vi "MotorSimulation.vi"() -> ()   [LabVIEW 2022 SP3]
panel:
  out "Input and theta":cluster{"Signal Gen":dbl, "Thetadot Out":dbl}(graph)
  in  "System Parameters":cluster{"a1":dbl, "a0":dbl, "a2 ":dbl, "b":dbl}={"a1"=0.1894, "a0"=0.0, "a2 "=0.0052, "b"=0.3334}
  in  "Ring":u16(ring) items=["square", "triangle", "sinusoidal"]
  in  "stop":bool
  out "Input and thetadot":cluster{"Signal Gen":dbl, "Thetadot Out":dbl}(graph)
  in  "Amplitude":dbl
  in  "Signal Freq (Hz)":dbl
  in  "Sampling Time  (s)":dbl
  # "Lab 2"
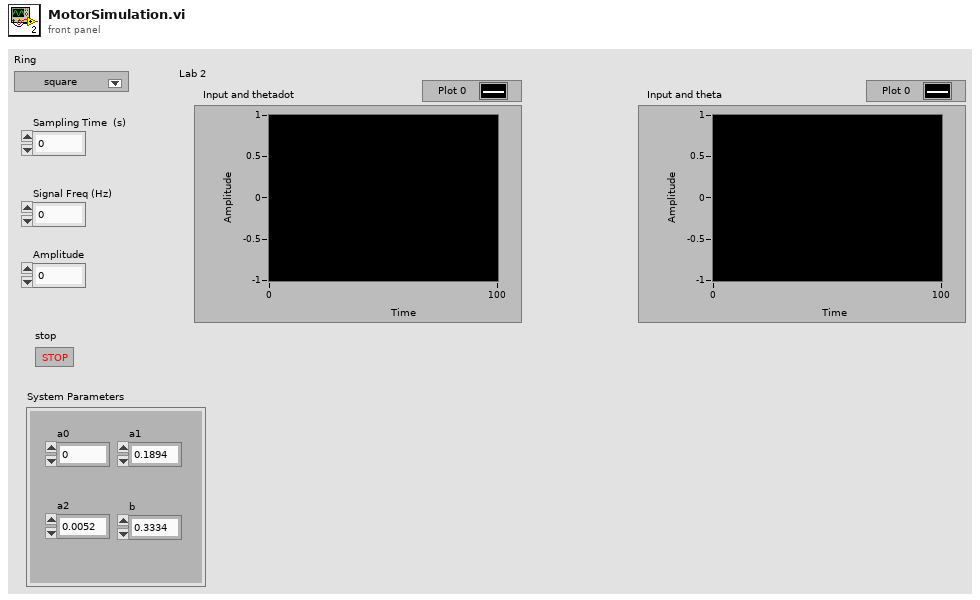
[diagram p1: front panel]
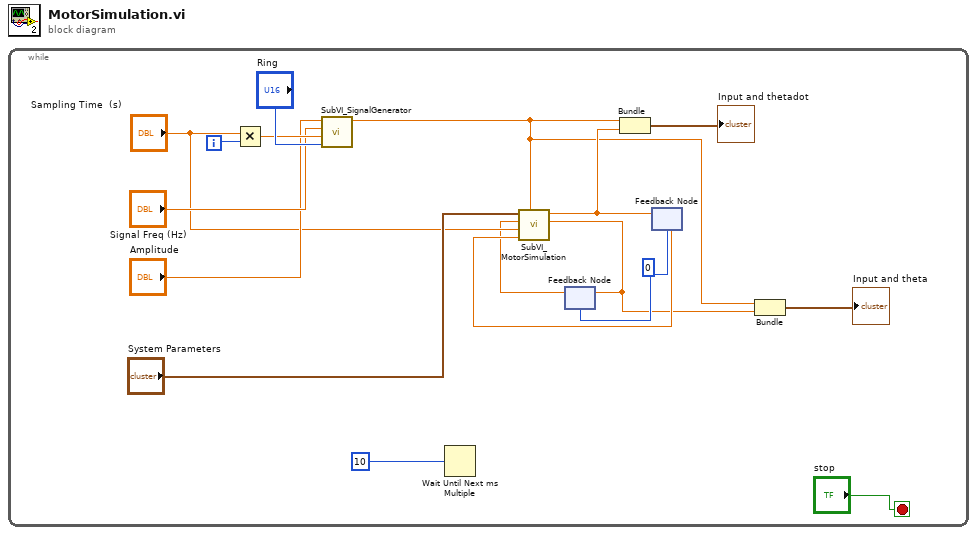
[diagram p0: block diagram]
diagram:
  n1 = while {
    i -> [w15]
    stop <- "stop" stop-if-true
    w7 = 0
    n2 = Multiply(x="Sampling Time  (s)", y=w15) -> (x*y=w14:dbl)
    n3 = call "SubVI_SignalGenerator.vi"("Signal Type"="Ring", "Time"=w14, "Freq"="Signal Freq (Hz)", "Amplitude"="Amplitude") -> ("Signal Gen"=w4:dbl)  [unwired: 7 in]
    n4 = Wait Until Next ms Multiple(millisecond multiple=10) -> ()  [unwired: 1 out]
    n5 = feedback #1(w7) -> (w8:dbl)
    n6 = feedback #2(w7) -> (w9:dbl)
    n7 = call "SubVI_MotorSimulation.vi"("Input Voltage"=w4, "Velocity Reading"=w9, "dt [s]"="Sampling Time  (s)", "Position Reading"=w8, "System Parameters"="System Parameters") -> ("Theta Out"=w3:dbl, "Thetadot Out"=w6:dbl)  [unwired: 5 in]
    n8 = feedback-in #1(w3) -> ()
    n9 = Bundle("Signal Gen"=w4, "Thetadot Out"=w6) -> (→"Input and thetadot":cluster{"Signal Gen":dbl, "Thetadot Out":dbl})  [unwired: 1 in]
    n10 = feedback-in #2(w6) -> ()
    n11 = Bundle("Signal Gen"=w4, "Theta Out"=w3) -> (→"Input and theta":cluster{"Signal Gen":dbl, "Theta Out":dbl})  [unwired: 1 in]
  }
